vi "Read Default Value.vi"(8 "error in (no error)":errorcluster, 11 "String Data Type in":refnum<class "String Data Type.lvclass">) -> (0 "error out":errorcluster, 2 "Default Value":string, 3 "String Data Type out":refnum<class "String Data Type.lvclass">)   [LabVIEW 2018, in "String Data Type.lvclass"]
uses:
  String Data Type.lvclass
  String Data Type.lvclass/String Data Type.ctl
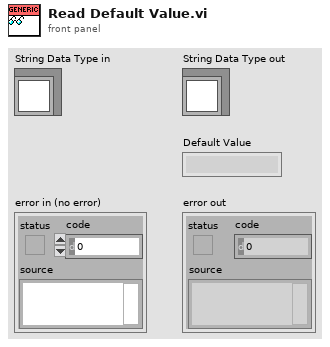
[diagram p1: front panel]
types:
  T1 = typedef "String Data Type.lvclass/Display Style Enum.ctl" = enum16{"Normal", "'\\' Codes", "Hex"}
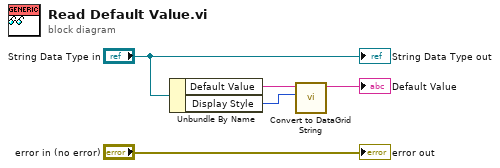
[diagram p0: block diagram]
diagram:
  n1 = Unbundle By Name("String Data Type in") -> ("Default Value"=w3:string, "Display Style"=w2:T1)
  n2 = call "Convert to DataGrid String.vi"("Display Style"=w2, "Popup String in"=w3) -> ("DataGrid String out"=→"Default Value":string)  [unwired: 9 in]
  "error out" <- "error in (no error)"
  "String Data Type out" <- "String Data Type in"
